vi "Unit_value_maps.vi"(10 "UNIT":string, 11 "Actual String":string) -> (3 "Actual value":dbl)   [LabVIEW 2024, in "Test_2.lvlib"]
uses:
  Test_2.lvlib
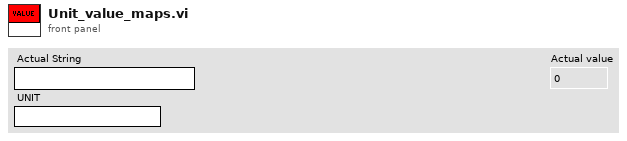
[diagram p1: front panel]
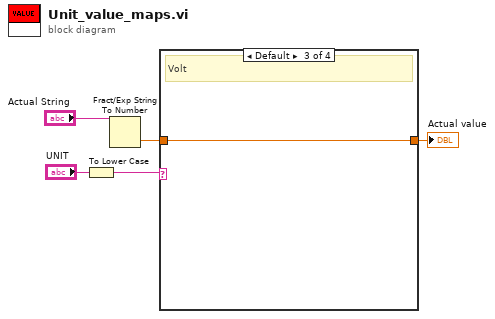
[diagram p0: block diagram]
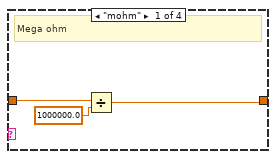
[diagram p2: hidden frame]
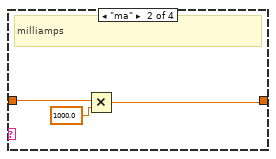
[diagram p3: hidden frame]
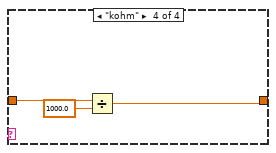
[diagram p4: hidden frame]
diagram:
  n1 = To Lower Case(string="UNIT") -> (all lower case string=w4:string)
  n2 = Fract/Exp String To Number(string="Actual String") -> (number=w2:dbl)  [unwired: 3 in, 1 out]
  n3 = case shown="Default" w4 {
    tunnel: w2 -> [w8 w11 w12 w15]
    tunnel: [w6 w9 w12 w13] -> w1
    frame "mohm" {
      # "Mega ohm"
      n4 = Divide(x=w8, y=1000000.0) -> (x/y=w6:dbl)
    }
    frame "ma" {
      # "milliamps"
      n5 = Multiply(x=w11, y=1000.0) -> (x*y=w9:dbl)
    }
    frame Default {
      # "Volt"
    }
    frame "kohm" {
      n6 = Divide(x=w15, y=1000.0) -> (x/y=w13:dbl)
    }
  }
  "Actual value" <- w1
